vi "ALTS-2015 LV2GBL Task Pass Status.vi"(7 "Options":T1(ring)=enum."Set Task Pass", 8 "error in":errorcluster, 10 "Task Failure State in":bool=TRUE, 11 "Task Pass State in":bool=TRUE) -> (0 "error out":errorcluster, 2 "Task Failure State Out":bool, 3 "Task Pass State Out":bool)   [LabVIEW 2013]
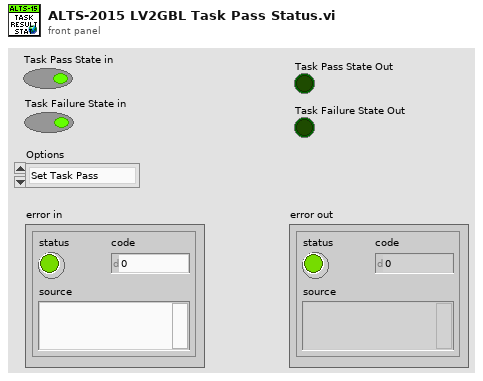
[diagram p1: front panel]
types:
  T1 = enum16{"Init", "Set Task Pass", "Set Task Failure", "Set Task Status", "Get"}
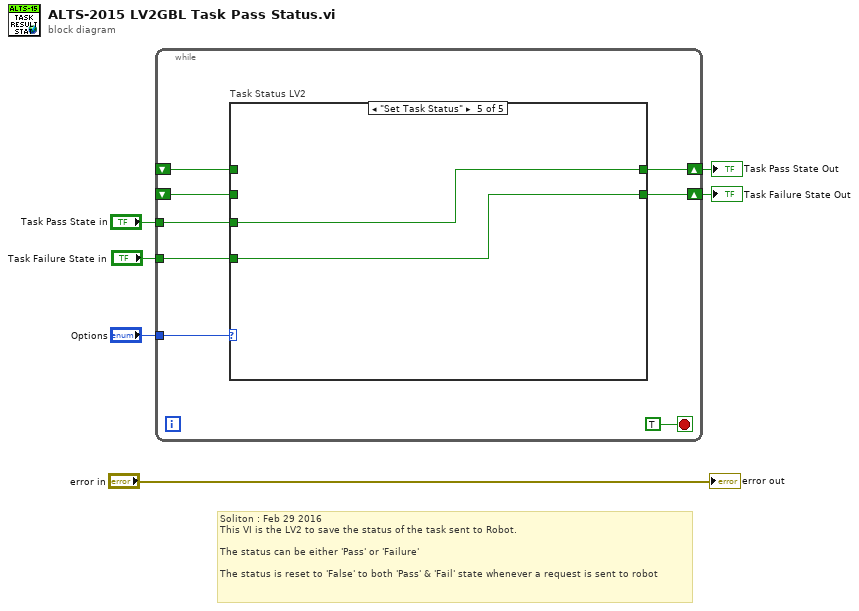
[diagram p0: block diagram]
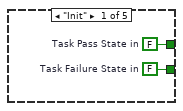
[diagram p2: hidden frame]
diagram:
  # "Soliton : Feb 29 2016\nThis VI is the LV2 to save the status of the task sent to Robot.\n\nThe status can be either 'Pass' or 'Failure'\n\nThe status is reset to 'False' to both 'Pass' & 'Fail' state whenever a request is sent to robot"
  n1 = while {
    tunnel: "Options" -> [w14]
    tunnel: "Task Pass State in" -> [w12]
    shift-right: [w13] -> w4
    shift-left: _ -> [w11]
    tunnel: "Task Failure State in" -> [w9]
    shift-right: [w8] -> w1
    shift-left: _ -> [w7]
    stop <- TRUE stop-if-true
    n2 = case "Task Status LV2" shown="\"Set Task Status\"" w14 {
      tunnel: [w16 w18 w20 w21 w24] -> w13
      tunnel: w12 -> [_ _ w20 _ w24]
      tunnel: w11 -> [_ w18 _ w21 _]
      tunnel: w9 -> [_ _ _ w22 w23]
      tunnel: [w15 w17 w19 w22 w23] -> w8
      tunnel: w7 -> [_ w17 w19 _ _]
      frame "Init" {
        w15 = FALSE  # Task Failure State in
        w16 = FALSE  # Task Pass State in
      }
      frame "Get" {
      }
      frame "Set Task Pass" {
      }
      frame "Set Task Failure" {
      }
      frame "Set Task Status" {
      }
    }
  }
  "Task Pass State Out" <- w4
  "Task Failure State Out" <- w1
  "error out" <- "error in"
